vi "Handle.vi"(11 "jettl Queue Actor in":refnum<class "jettl Queue Actor.lvclass">) -> (2 "Destroy?":bool, 3 "jettl Queue Actor out":refnum<class "jettl Queue Actor.lvclass">)   [LabVIEW 2021, in "jettl.lvlib" / "jettl Queue Actor.lvlib" / "jettl Queue Actor.lvclass"]
uses:
  jettl Queue Actor.lvclass
  C:/git/jettl/src/Actor/Queue Actor/Queue Actor.lvclass
  jettl Queue Actor.lvclass/jettl Queue Actor.ctl
  State/State/State.lvclass
  jettl.lvlib
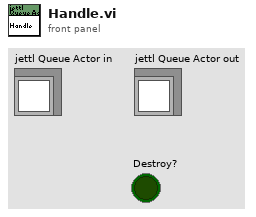
[diagram p1: front panel]
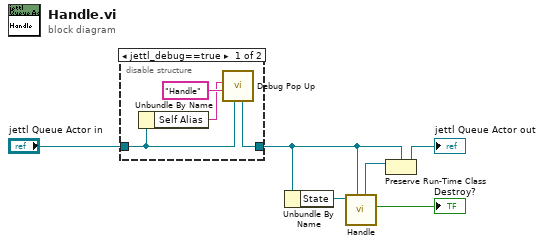
[diagram p0: block diagram]
diagram:
  n1 = disable-structure shown="jettl_debug==true" {
    disable-tunnel: "jettl Queue Actor in" -> [w8 _]
    disable-tunnel: [w9 _] -> w2
    frame condition #0 (active) {
      n2 = Unbundle By Name(w8) -> ("Self Alias"=w7:string)
      n3 = call "Debug Pop Up.vi"("Input"=w8, "Method"="Handle", "Alias"=w7) -> ("Output"=w9:refnum<class "jettl Queue Actor.lvclass">)  [unwired: 8 in]
    }
    frame condition #1 {
    }
  }
  n4 = Unbundle By Name(w2) -> ("State"=w6:refnum<class "State.lvclass">)
  n5 = call-dynamic "Handle.vi"("Queue Actor in"=w2, "State in"=w6) -> ("Destroy?"=→"Destroy?":bool, "Queue Actor out"=w4:refnum<class "Queue Actor.lvclass">)  [unwired: 8 in]
  n6 = Preserve Run-Time Class(object in=w4, 2:w2) -> (object out=→"jettl Queue Actor out":refnum<class "jettl Queue Actor.lvclass">)  [unwired: 1 in, 1 out]
